vi "_PC_Pub_Memory_Pressure.vi"(7 "Function":enum16{"Init", "Write", "Read"}(ring)=enum."Read", 8 "error in (no error)":errorcluster, 10 "Pressure in":dbl) -> (0 "error out":errorcluster, 2 "Pressures":dbl[](array[numeric]))   [LabVIEW 2018]
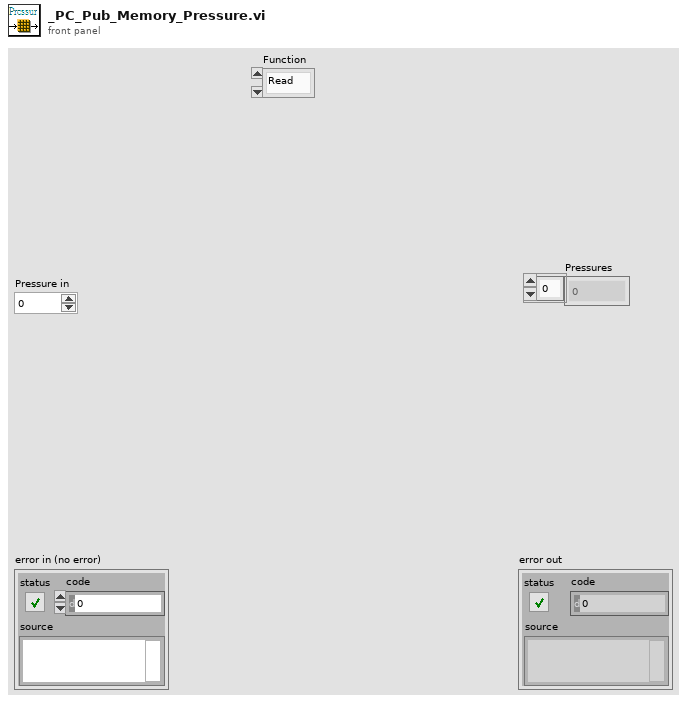
[diagram p1: front panel]
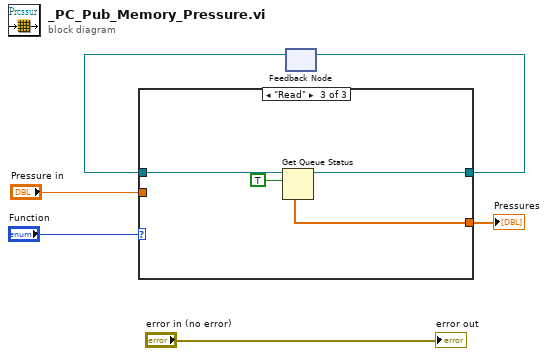
[diagram p0: block diagram]
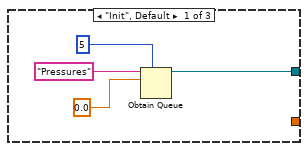
[diagram p2: hidden frame]
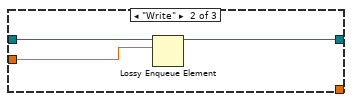
[diagram p3: hidden frame]
diagram:
  n1 = feedback #1() -> (w4:refnum<queue>)  [unwired: 1 in]
  n2 = case shown="\"Read\"" "Function" {
    tunnel: [w9 w12 w16] -> w5
    tunnel: w4 -> [_ w13 w17]
    tunnel: "Pressure in" -> [_ w11 _]
    tunnel: [_ _ w14] -> w2
    frame "Init", Default {
      n3 = Obtain Queue(max queue size (-1, unlimited)=5, name (unnamed)="Pressures", element data type=0.0) -> (queue out=w9:refnum<queue>)  [unwired: 2 in, 2 out]
    }
    frame "Write" {
      n4 = Lossy Enqueue Element(queue=w13, element=w11) -> (queue out=w12:refnum<queue>)  [unwired: 1 in, 3 out]
    }
    frame "Read" {
      n5 = Get Queue Status(queue=w17, return elements? (F)=TRUE) -> (queue out=w16:refnum<queue>, elements=w14:dbl[])  [unwired: 1 in, 6 out]
    }
  }
  "Pressures" <- w2
  n6 = feedback-in #1(w5) -> ()
  "error out" <- "error in (no error)"
